vi "Quadratic_Equation.vi"() -> ()   [LabVIEW 2024]
panel:
  out "String 6":string
  in  "String 5":string
  in  "String 4":string
  out "String 3":string
  in  "String 2":string
  in  "String":string
  out "output variable 2":cxt
  out "output variable":cxt
  in  "input variable 3":dbl
  in  "input variable 2":dbl
  in  "input variable":dbl
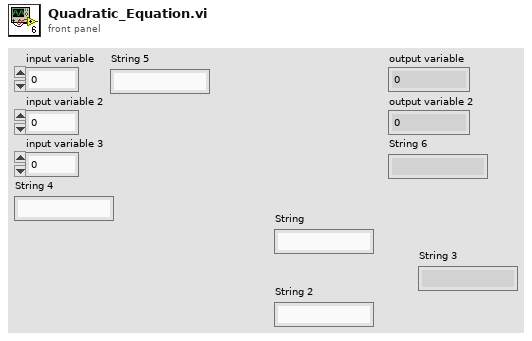
[diagram p1: front panel]
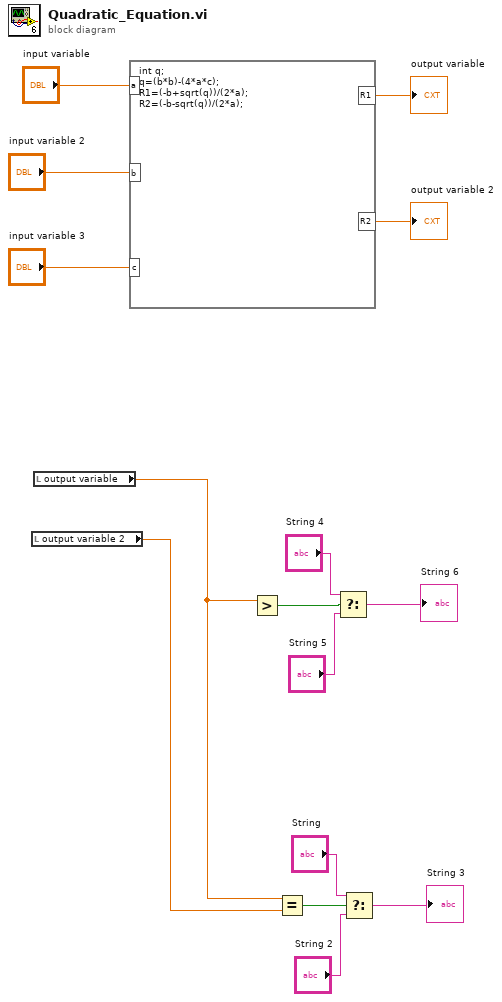
[diagram p0: block diagram]
diagram:
  n1 = local read "output variable 2"() -> (w3:cxt)
  n2 = local read "output variable"() -> (w2:cxt)
  n3 = formula code="int q;\nq=(b*b)-(4*a*c);\nR1=(-b+sqrt(q))/(2*a);\nR2=(-b-sqrt(q))/(2*a);"("a"="input variable", "b"="input variable 2", "c"="input variable 3") -> ("R1"=→"output variable":dbl, "R2"=→"output variable 2":dbl)
  n4 = Greater?(x=w2) -> (0:w1:bool)  [unwired: 1 in]
  n5 = Equal?(x=w2, y=w3) -> (x = y?=w10:bool)
  n6 = Select(t="String 4", s=w1, f="String 5") -> (s? t:f=→"String 6":string)
  n7 = Select(t="String", s=w10, f="String 2") -> (s? t:f=→"String 3":string)
